vi "NT0-Main.vi"() -> ()   [LabVIEW 2019]
uses:
  <vilib>/Rock Robotics/Network Tables/NT Globals.vi
  <vilib>/Rock Robotics/Network Tables/Manage Connection List.vi
  <vilib>/Rock Robotics/Network Tables/NT Read Boolean.vi
  <vilib>/Rock Robotics/Network Tables/NT Read Boolean Array.vi
  <vilib>/Rock Robotics/Network Tables/NT Read Number.vi
  <vilib>/Rock Robotics/Network Tables/NT Read Numeric Array.vi
  <vilib>/Rock Robotics/Network Tables/NT Read String.vi
  <vilib>/Rock Robotics/Network Tables/NT Read String Array.vi
  <vilib>/Rock Robotics/Network Tables/NT Write String Array.vi
  <vilib>/Rock Robotics/Network Tables/NT Write String.vi
  <vilib>/Rock Robotics/Network Tables/NT Write Numeric Array.vi
  <vilib>/Rock Robotics/Network Tables/NT Write Number.vi
  <vilib>/Rock Robotics/Network Tables/NT Write Boolean Array.vi
  <vilib>/Rock Robotics/Network Tables/NT Write Boolean.vi
panel:
  in  "DeleteAll":bool
  in  "DeleteNew":bool
  in  "CreateNew":bool
  in  "FlusehTest0":bool
  out "Connection Count":i32
  in  "Tab Control":enum32{"Info", "Test", "Tree"}(tab)
  out "Name":string
  out "Start Time":string
  out "Variable Count":i32
  out "ConnectionCount":i32
  out "IsClient":bool
  out "Produce Read Errors":bool
  out "ValidateTable":bool
  out "ConnectionNames":string[](array[string])
  out "InitComplete":bool[](array[boolean])
  out "Test-String":string
  out "Test-StringArray":string[](array[string])
  out "Test-NumbArray":dbl[](array[numeric])
  out "Test-BoolArray":bool[](array[boolean])
  out "Test-Bool":bool
  out "Test-Numb":dbl
  out "Tree":string(tree)
  out "Good3":bool
  out "Good2":bool
  out "Good1":bool
  out "Good0":bool
  out "Test3":dbl
  out "Test2":dbl
  out "Test1":dbl
  out "Test0":dbl
  out "NT Connection":bool
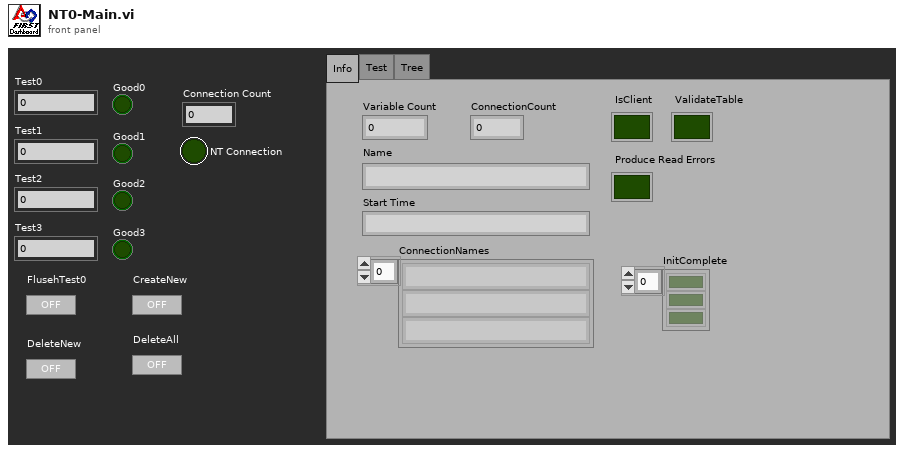
[diagram p1: front panel]
types:
  T1 = cluster{"Shift":bool, "Ctrl":bool, "Alt":bool, "Cmd":bool, "Opt":bool}
  T2 = typedef "LVDateTimeRec.ctl" = cluster{"fractional second":dbl, "second":i32, "minute":i32, "hour":i32, "day of month":i32, "month":i32, "year":i32, "day of week":i32, "day of year":i32, "DST":i32}
  T3 = typedef "ClientNTTestConfig.ctl" = cluster{"Elapsed0":string, "Name0":string, "Test0":u32, "Ellapsed1":string, "Name1":string, "Test1":u32, "Elapsed2":string, "Name2":string, "Test2":u32, "Elapsed3":string, "Name3":string, "Test3":u32, "NewName":string}
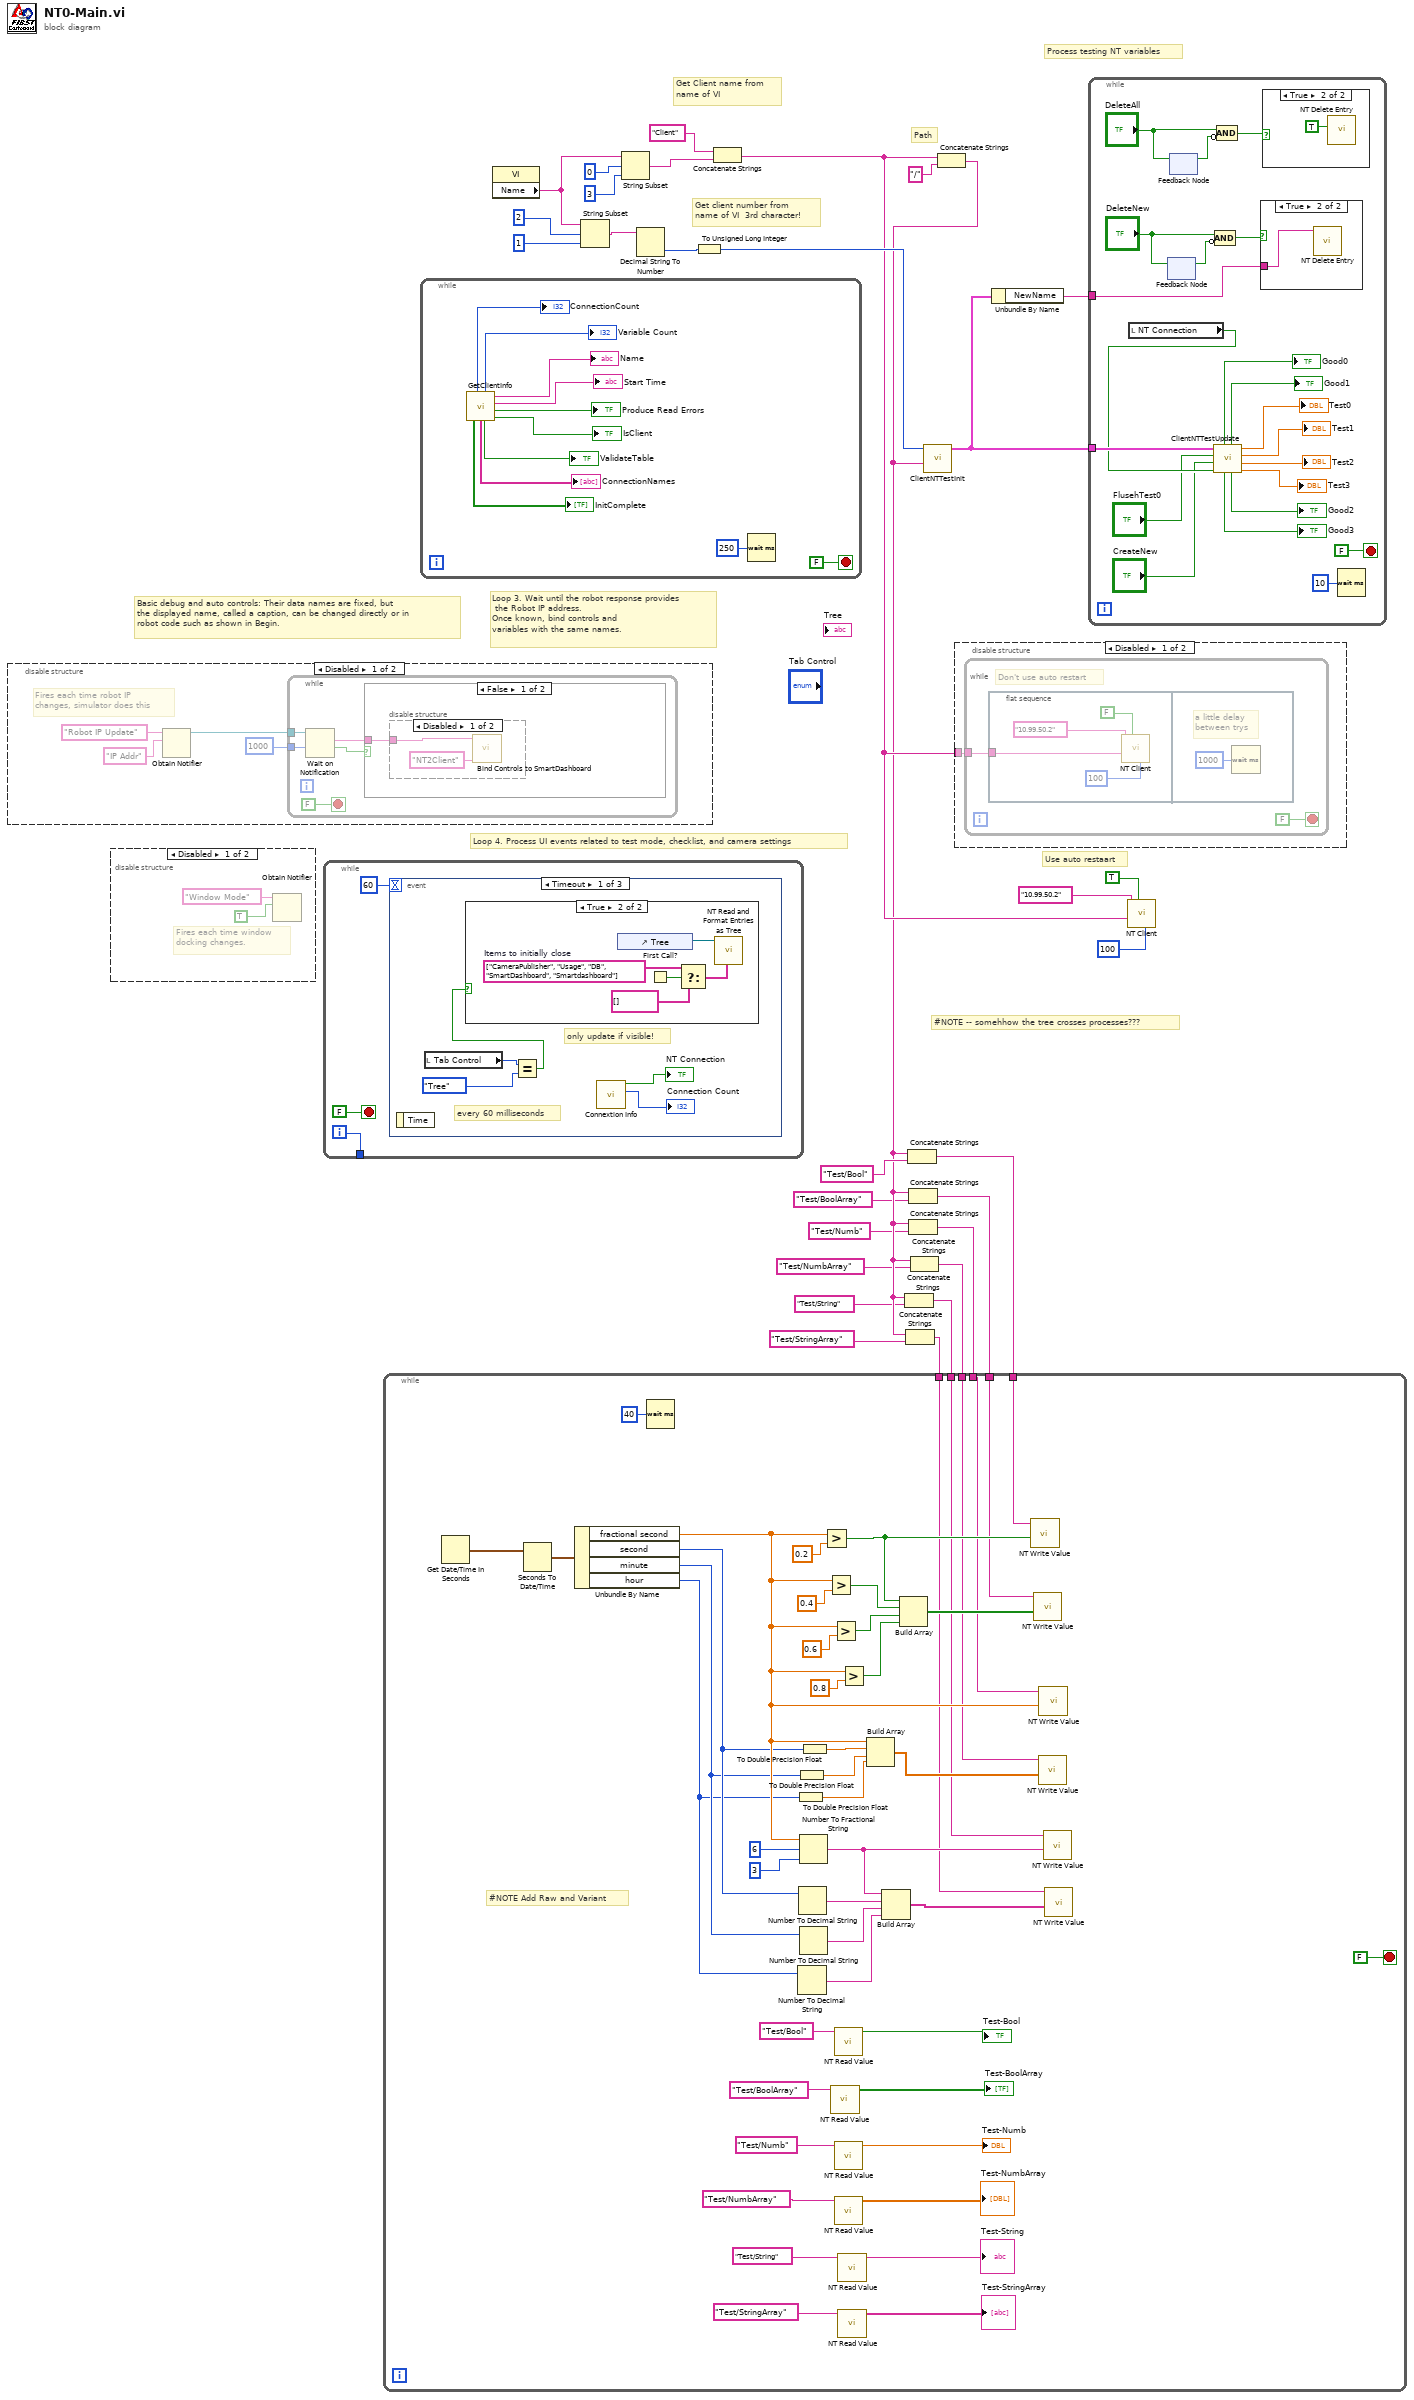
[diagram p0: block diagram]
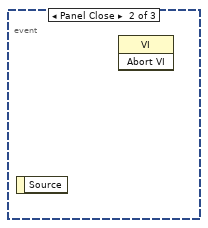
[diagram p10: hidden frame]
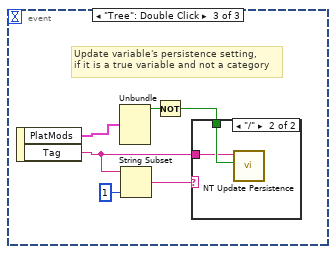
[diagram p11: hidden frame]
diagram:
  # "Path"
  # "Get Client name from\nname of VI"
  # "Get client number from\nname of VI  3rd character!"
  # "Process testing NT variables"
  # "Use auto restaart"
  # "#NOTE -- somehhow the tree crosses processes???"
  # "Basic debug and auto controls: Their data names are fixed, but\nthe displayed name, called a caption, can be changed directly or in\nrobot code such as shown in Begin."
  # "Loop 4. Process UI events related to test mode, checklist, and camera settings"
  # "Loop 3. Wait until the robot response provides\n the Robot IP address.\nOnce known, bind controls and\nvariables with the same names."
  n1 = disable-structure shown="Disabled" {
    frame Disabled {
      # "Fires each time robot IP\nchanges, simulator does this"
      n2 = Obtain Notifier(name (unnamed)="Robot IP Update", notification data type="IP Addr" ("name (unnamed)")) -> (notifier out=w31:refnum<notifier>)  [unwired: 2 in, 2 out]
      n3 = while {
        tunnel: w31 -> [w38]
        tunnel: u32 1000 ("milliseconds to wait") -> [w36]
        stop <- FALSE stop-if-true
        n4 = Wait on Notification(notifier=w38, timeout in ms (-1)=w36) -> (notification=w37:string, timed out?=w35:bool)  [unwired: 2 in, 2 out]
        n5 = case shown="False" w35 {
          tunnel: w37 -> [w40 _]
          frame False {
            n6 = disable-structure shown="Disabled" {
              disable-tunnel: w40 -> [w42 _]
              frame Disabled {
                n7 = call <vilib>:"Bind Controls to SmartDashboard.vi"("Client Name"="NT2Client", "Server IP Address"=w42) -> ()  [unwired: 10 in]
              }
              frame Enabled {
              }
            }
          }
          frame True {
          }
        }
      }
    }
    frame Enabled {
    }
  }
  n8 = disable-structure shown="Disabled" {
    frame Disabled {
      # "Fires each time window\ndocking changes."
      n9 = Obtain Notifier(name (unnamed)="Window Mode", notification data type=TRUE) -> ()  [unwired: 2 in, 3 out]
    }
    frame Enabled {
    }
  }
  n10 = while {
    tunnel: [w45] -> _
    i -> [w45]
    stop <- FALSE stop-if-true
    n11 = event shown="[0] Timeout" {
      selector: _ -> [_ _ _]
      dyn-events: _ -> [_ _ _]
      timeout: u32 60 ("milliseconds to wait") -> [_ _ _]
      event Timeout {
        # "only update if visible!"
        # "every 60 milliseconds"
        n12 = event-data() -> ()  [unwired: 1 in, 1 out]
        n13 = local read "Tab Control"() -> (w50:enum32{"Info", "Test", "Tree"})
        n14 = Equal?(x=w50, y=enum32{"Info", "Test", "Tree"}."Tree") -> (x = y?=w49:bool)
        n15 = case shown="True" w49 {
          frame False {
          }
          frame True {
            w57 = string[] ["CameraPublisher", "Usage", "DB", "SmartDashboard", "Smartdashboard"]  # Items to initially close
            n16 = control-ref of="Tree"() -> (w55:refnum<vi>)
            n17 = First Call?() -> (First Call?: T/F=w54:bool)
            n18 = Select(t=w57, s=w54, f=string[] []) -> (s? t:f=w53:string[])
            n19 = call <vilib>:"NT Read and Format Entries as Tree.vi"("Tags to  Close"=w53, "Tree Refnum"=w55) -> ()  [unwired: 8 in, 2 out]
          }
        }
        n20 = call <vilib>:"Connextion Info.vi"() -> ("Connection Count"=→"Connection Count":i32, "Connected"=→"NT Connection":bool)  [unwired: 10 in]
      }
      event Panel Close {
        n21 = event-data() -> ()  [unwired: 1 in, 1 out]
        n22 = invoke class="VI" method="Abort VI"() -> ()  [unwired: 3 in, 3 out]
      }
      event "Tree": Double Click {
        # "Update variable's persistence setting,\nif it is a true variable and not a category"
        n23 = event-data() -> ("PlatMods"=w59:T1, "Tag"=w58:string)  [unwired: 1 in]
        n24 = Unbundle(w59) -> ("Shift"=w63:bool)  [unwired: 4 out]
        n25 = String Subset(string=w58, length (rest)=1 ("length (rest)")) -> (substring=w60:string)  [unwired: 1 in]
        n26 = Not(x=w63) -> (.not. x?=w62:bool)
        n27 = case shown="\"/\"" w60 {
          tunnel: w62 -> [_ w65]
          tunnel: w58 -> [_ w64]
          frame Default {
          }
          frame "/" {
            n28 = call <vilib>:"NT Update Persistence.vi"("Persistence"=w65, "Name"=w64) -> ()  [unwired: 9 in, 1 out]
          }
        }
      }
    }
  }
  n29 = while {
    stop <- FALSE stop-if-true
    n30 = call "GetClientInfo.vi"() -> ("IsClient"=→"IsClient":bool, "Produce Read Errors"=→"Produce Read Errors":bool, "Start Time"=→"Start Time":string, "Name"=→"Name":string, "ValidateTable"=→"ValidateTable":bool, "Variable Count"=→"Variable Count":i32, "ConnectionNames"=→"ConnectionNames":string[], "ConnectionCount"=→"ConnectionCount":i32, "InitComplete"=→"InitComplete":bool[])  [unwired: 3 in]
    n31 = Wait (ms)(milliseconds to wait=u32 250) -> ()  [unwired: 1 out]
  }
  n32 = property class="VI"() -> ("Name"=w21:string)  [unwired: 2 in, 2 out]
  n33 = String Subset(string=w21, offset (0)=2, length (rest)=1 ("length (rest)")) -> (substring=w25:string)
  n34 = String Subset(string=w21, offset (0)=0, length (rest)=3 ("length (rest)")) -> (substring=w18:string)
  n35 = Decimal String To Number(string=w25) -> (number=w24:i32)  [unwired: 2 in, 1 out]
  n36 = To Unsigned Long Integer(number=w24) -> (unsigned 32bit integer=w23:u32)
  n37 = Concatenate Strings("Client" ("string"), w18) -> (w15:string)
  n38 = Concatenate Strings(w15, "/" ("string")) -> (w11:string)
  n39 = Concatenate Strings(w11, "Test/String" ("Name")) -> (w3:string)
  n40 = Concatenate Strings(w11, "Test/StringArray" ("Name")) -> (w1:string)
  n41 = Concatenate Strings(w11, "Test/Bool" ("Name")) -> (w12:string)
  n42 = Concatenate Strings(w11, "Test/BoolArray" ("Name")) -> (w9:string)
  n43 = Concatenate Strings(w11, "Test/Numb" ("Name")) -> (w7:string)
  n44 = Concatenate Strings(w11, "Test/NumbArray" ("Name")) -> (w5:string)
  n45 = while {
    tunnel: w12 -> [w94]
    tunnel: w9 -> [w93]
    tunnel: w7 -> [w92]
    tunnel: w5 -> [w91]
    tunnel: w3 -> [w90]
    tunnel: w1 -> [w89]
    stop <- FALSE stop-if-true
    # "#NOTE Add Raw and Variant"
    n46 = Get Date/Time In Seconds() -> (seconds since 1Jan1904=w122:timestamp)
    n47 = Seconds To Date/Time(time stamp (now)=w122) -> (date time rec=w121:T2)  [unwired: 1 in]
    n48 = Unbundle By Name(w121) -> ("fractional second"=w105:dbl, "second"=w101:i32, "minute"=w100:i32, "hour"=w99:i32)
    n49 = Wait (ms)(milliseconds to wait=u32 40) -> ()  [unwired: 1 out]
    n50 = To Double Precision Float(number=w99) -> (double precision float=w107:dbl)
    n51 = To Double Precision Float(number=w100) -> (double precision float=w108:dbl)
    n52 = Number To Decimal String(number=w99) -> (decimal integer string=w96:string)  [unwired: 1 in]
    n53 = Number To Decimal String(number=w101) -> (decimal integer string=w98:string)  [unwired: 1 in]
    n54 = Number To Fractional String(number=w105, width (-)=i16 6, precision (6)=i16 3) -> (F-format string=w102:string)  [unwired: 1 in]
    n55 = Number To Decimal String(number=w100) -> (decimal integer string=w97:string)  [unwired: 1 in]
    n56 = To Double Precision Float(number=w101) -> (double precision float=w109:dbl)
    n57 = Greater?(x=w105, y=0.2) -> (0:w116:bool)
    n58 = Greater?(x=w105, y=0.4) -> (0:w115:bool)
    n59 = call-poly <vilib>:"NT Read Value.vi"("Name"="Test/BoolArray") -> ("Boolean Array"=→"Test-BoolArray":bool[])  [unwired: 9 in, 1 out]
    n60 = Greater?(x=w105, y=0.6) -> (0:w114:bool)
    n61 = call-poly <vilib>:"NT Read Value.vi"("Name"="Test/Bool") -> ("Boolean"=→"Test-Bool":bool)  [unwired: 9 in, 1 out]
    n62 = call-poly <vilib>:"NT Read Value.vi"("Name"="Test/Numb") -> ("Numeric"=→"Test-Numb":dbl)  [unwired: 9 in, 1 out]
    n63 = call-poly <vilib>:"NT Read Value.vi"("Name"="Test/NumbArray") -> ("Numeric Array"=→"Test-NumbArray":dbl[])  [unwired: 9 in, 1 out]
    n64 = call-poly <vilib>:"NT Read Value.vi"("Name"="Test/String") -> ("String"=→"Test-String":string)  [unwired: 9 in, 1 out]
    n65 = call-poly <vilib>:"NT Read Value.vi"("Name"="Test/StringArray") -> ("String Array"=→"Test-StringArray":string[])  [unwired: 9 in, 1 out]
    n66 = Greater?(x=w105, y=0.8) -> (0:w113:bool)
    n67 = Build Array(w105, w109, w108, w107) -> (w106:dbl[])
    n68 = Build Array(w102, w98, w97, w96) -> (w95:string[])
    n69 = Build Array(w116, w115, w114, w113) -> (w110:bool[])
    n70 = call-poly <vilib>:"NT Write Value.vi"("Boolean"=w116, "Name"=w94) -> ()  [unwired: 9 in, 1 out]
    n71 = call-poly <vilib>:"NT Write Value.vi"("Boolean Array"=w110, "Name"=w93) -> ()  [unwired: 9 in, 1 out]
    n72 = call-poly <vilib>:"NT Write Value.vi"("Numeric Array"=w106, "Name"=w91) -> ()  [unwired: 9 in, 1 out]
    n73 = call-poly <vilib>:"NT Write Value.vi"("Numeric"=w105, "Name"=w92) -> ()  [unwired: 9 in, 1 out]
    n74 = call-poly <vilib>:"NT Write Value.vi"("String"=w102, "Name"=w90) -> ()  [unwired: 9 in, 1 out]
    n75 = call-poly <vilib>:"NT Write Value.vi"("String Array"=w95, "Name"=w89) -> ()  [unwired: 9 in, 1 out]
  }
  n76 = call "ClientNTTestInit.vi"("Prefix"=w11, "Instance"=w23) -> ("TestConfig"=w17:T3)  [unwired: 9 in]
  n77 = disable-structure shown="Disabled" {
    disable-tunnel: w15 -> [w123 _]
    frame Disabled {
      n78 = while {
        tunnel: w123 -> [w124]
        stop <- FALSE stop-if-true
        # "Don't use auto restart"
        n79 = flat-sequence {
          tunnel: w124 -> [w126]
          frame #0 {
            n80 = call <vilib>:"NT Client.vi"("Update Time"=100, "Automatic restart"=FALSE, "Client Name"=w126, "Server IP Address"="10.99.50.2") -> ()  [unwired: 8 in]
          }
          frame #1 {
            # "a little delay\nbetween trys"
            n81 = Wait (ms)(milliseconds to wait=u32 1000) -> ()  [unwired: 1 out]
          }
        }
      }
    }
    frame Enabled {
    }
  }
  n82 = Unbundle By Name(w17) -> ("NewName"=w16:string)
  n83 = while {
    tunnel: w17 -> [w151]
    tunnel: w16 -> [w131]
    stop <- FALSE stop-if-true
    n84 = local read "NT Connection"() -> (w140:bool)
    n85 = feedback #1() -> (w135:bool)  [unwired: 1 in]
    n86 = feedback-in #1("DeleteNew") -> ()
    n87 = feedback-in #2("DeleteAll") -> ()
    n88 = feedback #2() -> (w136:bool)  [unwired: 1 in]
    n89 = call "ClientNTTestUpdate.vi"("NT Connection"=w140, "CreateTestNew"="CreateNew", "Flush0"="FlusehTest0", "TestConfig"=w151) -> ("Value3"=→"Test3":dbl, "Value2"=→"Test2":dbl, "Value1"=→"Test1":dbl, "Value0"=→"Test0":dbl, "Good2"=→"Good2":bool, "Good1"=→"Good1":bool, "Good3"=→"Good3":bool, "Good0"=→"Good0":bool)
    n90 = Compound Arithmetic op=AND("DeleteNew", invert w135) -> (w132:bool)
    n91 = Compound Arithmetic op=AND("DeleteAll", invert w136) -> (w137:bool)
    n92 = case shown="True" w132 {
      tunnel: w131 -> [_ w152]
      frame False {
      }
      frame True {
        n93 = call <vilib>:"NT Delete Entry.vi"("Name"=w152) -> ()  [unwired: 10 in, 1 out]
      }
    }
    n94 = case shown="True" w137 {
      frame False {
      }
      frame True {
        n95 = call <vilib>:"NT Delete Entry.vi"("All"=TRUE) -> ()  [unwired: 10 in, 1 out]
      }
    }
    n96 = Wait (ms)(milliseconds to wait=u32 10) -> ()  [unwired: 1 out]
  }
  n97 = call <vilib>:"NT Client.vi"("Update Time"=100, "Automatic restart"=TRUE, "Client Name"=w15, "Server IP Address"="10.99.50.2") -> ()  [unwired: 8 in]
